vi "TestM1M3ILCMessageCreationPerformance.vi"() -> ()   [LabVIEW 2016]
uses:
  Common_RT_Modbus/ModbusBuffer/ModbusBuffer.lvclass
  Common_RT_ILC/ILC/ILC.lvclass
  Common_RT_ILC/ILC/ILC.lvclass/ILC.ctl
  Common_RT_Modbus/ModbusBuffer/ModbusBuffer.lvclass/ModbusBuffer.ctl
  Common_RT_Modbus/ModbusBuffer/writeHeader.vi
  Common_RT_Modbus/ModbusBuffer/writeU8.vi
  Common_RT_Modbus/ModbusBuffer/writeU16.vi
  Common_RT_Modbus/ModbusBuffer/writeCRC.vi
  Common_RT_Modbus/ModbusBuffer/writeEndOfFrame.vi
  Common_RT_Modbus/ModbusBuffer/writeWaitForRx.vi
  Common_RT_Modbus/ModbusBuffer/writeByteInstruction.vi
  Common_RT_Modbus/ModbusBuffer/calculateCRC.vi
panel:
  out "Time (us)":u32
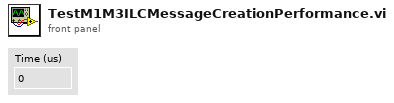
[diagram p1: front panel]
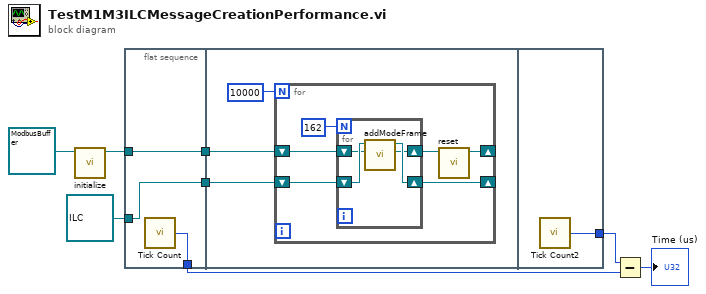
[diagram p0: block diagram]
diagram:
  n1 = call "initialize.vi"("ModbusBuffer in"=refnum<class "ModbusBuffer.lvclass"> refnum ("RTModbus.lvlib:ModbusBuffer.lvclass")) -> ("ModbusBuffer out"=w6:refnum<class "ModbusBuffer.lvclass">)  [unwired: 9 in, 1 out]
  n2 = flat-sequence {
    tunnel: [w11] -> w7
    tunnel: w6 -> [w11]
    tunnel: [w10] -> w5
    tunnel: refnum<class "ILC.lvclass"> refnum ("RTILC.lvlib:ILC.lvclass") -> [w10]
    tunnel: [w9] -> w2
    tunnel: w7 -> [w13]
    tunnel: w5 -> [w12]
    tunnel: [w25] -> w3
    frame #0 {
      n3 = call "Tick Count"() -> ("Tick Count(uSec)"=w9:u32)
    }
    frame #1 {
      n4 = for {
        N: 10000 -> [_]
        shift-right: [w16] -> _
        shift-left: w13 -> [w19]
        shift-right: [w15] -> _
        shift-left: w12 -> [w20]
        n5 = for {
          N: 162 -> [_]
          shift-right: [w23] -> w15
          shift-left: w20 -> [w24]
          shift-right: [w22] -> w17
          shift-left: w19 -> [w21]
          n6 = call "addModeFrame.vi"("ModbusBuffer in"=w21, "ILC in"=w24) -> ("ModbusBuffer out"=w22:refnum<class "ModbusBuffer.lvclass">, "ILC out"=w23:refnum<class "ILC.lvclass">)  [unwired: 7 in, 1 out]
        }
        n7 = call "reset.vi"("ModbusBuffer in"=w17) -> ("ModbusBuffer out"=w16:refnum<class "ModbusBuffer.lvclass">)  [unwired: 9 in, 1 out]
      }
    }
    frame #2 {
      n8 = call "Tick Count2"() -> ("Tick Count(uSec)"=w25:u32)
    }
  }
  n9 = Subtract(x=w3, y=w2) -> (x-y=→"Time (us)":u32)
